vi "TankFillLevelSafety.vi"(0 "pump":bool, 1 "enable":bool, 5 "tank":bool, 7 "intlet valve":bool, 9 "outlet valve":bool, 11 "fill level t-1":dbl, 12 "fill level t-2":dbl) -> (3 "pump":bool, 4 "outlet valve":bool, 6 "max level t-1":bool, 8 "inlet valve":bool, 10 "min level t-1":bool, 14 "min level t-2":bool, 15 "max level t-2":bool)   [LabVIEW 2011]
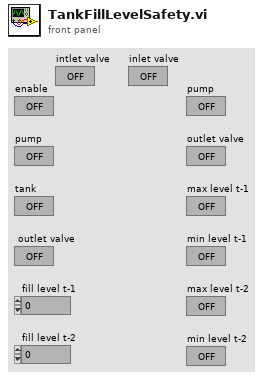
[diagram p1: front panel]
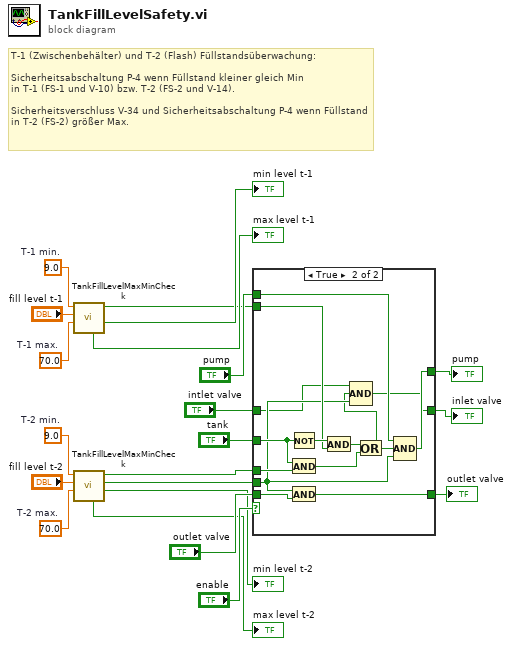
[diagram p0: block diagram]
diagram:
  w3 = 70.0  # T-2 max.
  w13 = 70.0  # T-1 max.
  w8 = 9.0  # T-2 min.
  w10 = 9.0  # T-1 min.
  # "T-1 (Zwischenbehälter) und T-2 (Flash) Füllstandsüberwachung:\n\nSicherheitsabschaltung P-4 wenn Füllstand kleiner gleich Min\nin T-1 (FS-1 und V-10) bzw. T-2 (FS-2 und V-14).\n\nSicherheitsverschluss V-34 und Sicherheitsabschaltung P-4 wenn Füllstand in T-2 (FS-2) größer Max."
  n1 = call "TankFillLevelMaxMinCheck.vi"("max level"=w13, "fill level"="fill level t-1", "min level"=w10) -> ("below min"=→"min level t-1":bool, "over min"=w11:bool, "over max"=→"max level t-1":bool)  [unwired: 5 in, 1 out]
  n2 = call "TankFillLevelMaxMinCheck.vi"("max level"=w3, "fill level"="fill level t-2", "min level"=w8) -> ("below min"=→"min level t-2":bool, "below max"=w5:bool, "over min"=w6:bool, "over max"=→"max level t-2":bool)  [unwired: 5 in]
  n3 = case shown="True" "enable" {
    tunnel: w6 -> [_ w36]
    tunnel: w11 -> [_ w35]
    tunnel: w5 -> [_ w28]
    tunnel: [w24 w33] -> w16
    tunnel: [w23 w32] -> w17
    tunnel: "pump" -> [w24 w31]
    tunnel: "outlet valve" -> [w23 w30]
    tunnel: "tank" -> [_ w29]
    tunnel: [w22 w25] -> w2
    tunnel: "intlet valve" -> [w22 w26]
    frame False {
    }
    frame True {
      n4 = Not(x=w29) -> (.not. x?=w38:bool)
      n5 = And(x=w29, y=w36) -> (x .and. y?=w37:bool)
      n6 = And(x=w28, y=w30) -> (x .and. y?=w32:bool)
      n7 = And(x=w38, y=w35) -> (x .and. y?=w34:bool)
      n8 = Or(x=w34, y=w37) -> (x .or. y?=w27:bool)
      n9 = Compound Arithmetic op=AND(w26, w27, w28) -> (w25:bool)
      n10 = Compound Arithmetic op=AND(w31, w27, w28) -> (w33:bool)
    }
  }
  "outlet valve" <- w17
  "pump" <- w16
  "inlet valve" <- w2
